vi "HEWH Trigger Below Setpoint.vi"(5 "Station D":T1={"Sequence #"=0.0, "Cycles"=0, "Mode Setting"="", "Flow Rate (GPM)"=0.0, "Temperature (F)"=0.0, "Reset Timer"=FALSE, "Use Temp Decline Method"=FALSE, "Terminate Condition"=enum."C1-Terminate Draw @ Gallon Mark", "Condition Value #1"=0.0, "UE"=FALSE, "LE"=FALSE, "Comp"=FALSE, "Fan"=FALSE, "Test End Time (Sec)"=0.0, "Purge Until Cutout"=FALSE, "Start Conditions"=enum."Heat Source Cutout", "Condition Value #2"=0.0, "Remove Power"=FALSE, "Time"=0.0, "Check Special Cond."=enum."SC2-Check Heat Source (On-C2/Off-C1)", "Condition#"=enum."C1", "Draw Flags"=enum."N/A", "Data Processing Delay (FHD 15sec, UEF 5 Sec)"=0.0, "Test Complete"=FALSE} {"Time" format="%<%H:%M:%S>t"}, 7 "Full Cutout":bool, 8 "Error In":errorcluster, 9 "Array Index":i32, 10 "TC Tree Array":dbl[](array[numeric]), 11 "StationA Setpoint":i32=140 caption="Unit Setpoint") -> (0 "Error Out":errorcluster, 3 "Trigger Draw":bool)   [LabVIEW 2016]
uses:
  Type Definitions/PRAT Test.ctl
  Utility/Save File/File Setup (Public)/Type Definition/Save File HEWH Heating Control Mode.ctl
  Draw Water Specific/Type Definitions/Terminate Draw Conditions.ctl
  Type Definitions/HEWH Start Conditions.ctl
  Draw Water Specific/Type Definitions/Check Special Condtions.ctl
  Draw Water Specific/Type Definitions/HEWH Special Condition Check.ctl
  Type Definitions/HEWH Draw Flag ENUM.ctl
  Utility/Custom Pallet Controls/Custom Pallet String.ctl
  Utility/Type Definitions/UTILITY Notifier.ctl
  Utility/Save File/File Setup.lvlib
panel:
  out "Selected TC Temp (°F)":dbl
  out "Draw Until Temp (°F)":dbl
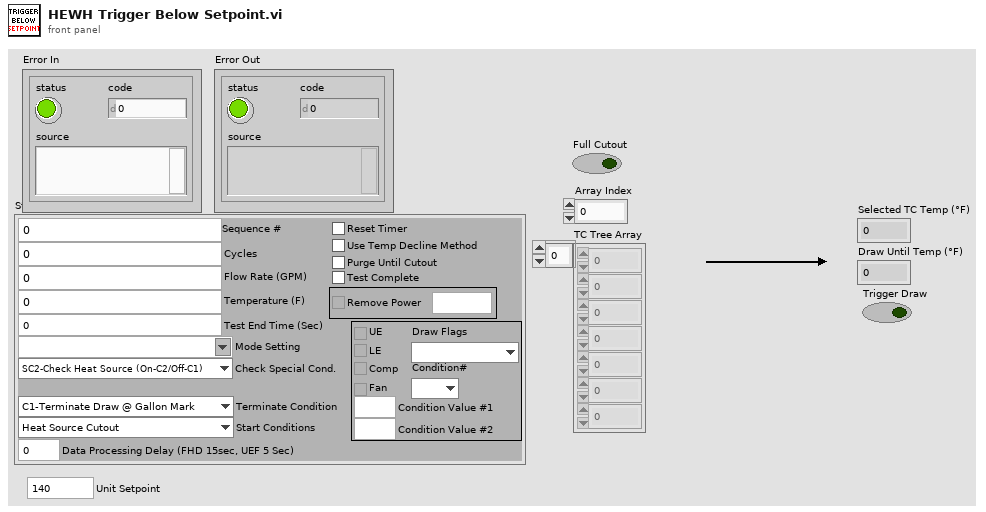
[diagram p1: front panel]
types:
  T1 = typedef "PRAT Test.ctl" = cluster{"Sequence #":dbl, "Cycles":i32, "Mode Setting":T2, "Flow Rate (GPM)":dbl, "Temperature (F)":dbl, "Reset Timer":bool, "Use Temp Decline Method":bool, "Terminate Condition":T3, "Condition Value #1":dbl, "UE":bool, "LE":bool, "Comp":bool, "Fan":bool, "Test End Time (Sec)":dbl, "Purge Until Cutout":bool, "Start Conditions":T4, "Condition Value #2":dbl, "Remove Power":bool, "Time":dbl, "Check Special Cond.":T5, "Condition#":T6, "Draw Flags":T7, "Data Processing Delay (FHD 15sec, UEF 5 Sec)":dbl, "Test Complete":bool}
  T2 = typedef "File Setup.lvlib/Save File HEWH Heating Control Mode.ctl" = string
  T3 = typedef "Terminate Draw Conditions.ctl" = enum16{"C1-Terminate Draw @ Gallon Mark", "C2-Special Last Draw (HU Test)", "C3-RTD Out <=", "C4-Mean Tank Temp <=", "C5-Decrease RTD Out (Deg F)", "C6-Time (Seconds)", "C7-Until Any Heat Source", "C8-Specific Heat Source", "C9-Do Nothing"}
  T4 = typedef "HEWH Start Conditions.ctl" = enum16{"Heat Source Cutout", "At Time (Seconds)", "Every X (Seconds)", "T2 >= X° Below Setpoint", "Seconds From Complete", "Wait for LE & Comp Cutout", "Wait for Comp Cutout", "Wait for LE Cutout", "Wait for UE Cutout"}
  T5 = typedef "Check Special Condtions.ctl" = enum16{"SC1-Do Nothing", "SC2-Check Heat Source (On-C2/Off-C1)", "SC3-Check Skip Condition", "SC4-Check Heat Source ON/Fail"}
  T6 = typedef "HEWH Special Condition Check.ctl" = enum16{"N/A", "C1", "C2", "Reset/Fail", "Skip Draw Sequence"}
  T7 = typedef "HEWH Draw Flag ENUM.ctl" = enum16{"N/A", "None(0)", "Sml(1)", "Med(2)", "SmlMed(3)", "Lrg(4)", "SmlLrg(5)", "MedLrg(6)", "SmlMedLrg(7)"}
  T8 = typedef "Custom Pallet String.ctl" = string
  T9 = typedef "UTILITY Notifier.ctl" = enum16{"Set", "Read", "Release Ref"}
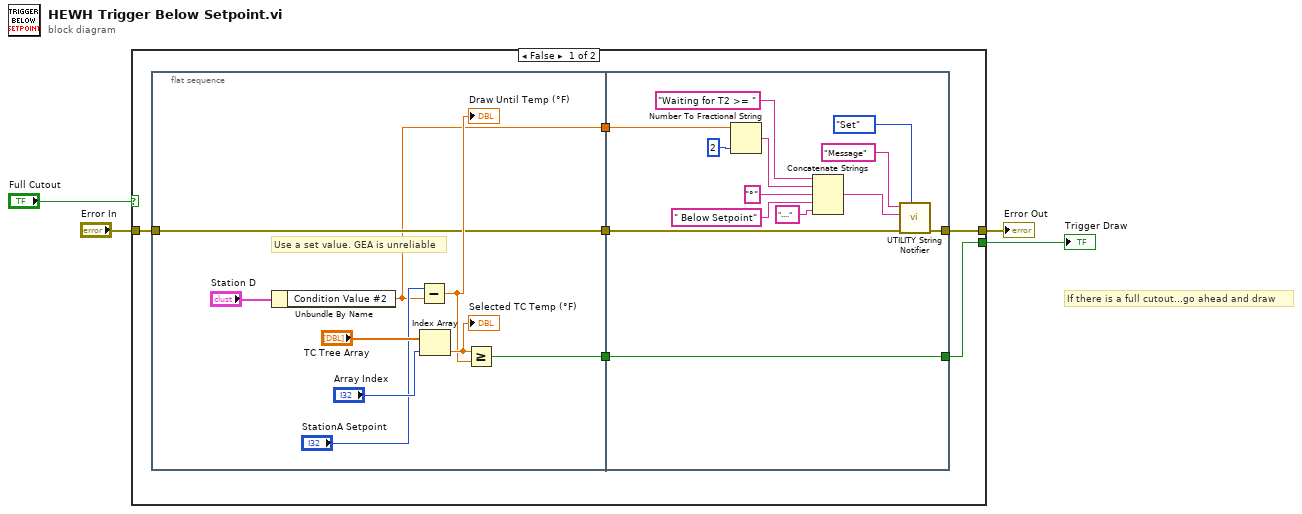
[diagram p0: block diagram]
diagram:
  # "If there is a full cutout...go ahead and draw"
  n1 = case shown="False" "Full Cutout" {
    selector: "Full Cutout" -> [_ w34]
    tunnel: [w10 w34] -> w4
    tunnel: "Error In" -> [w8 w33]
    tunnel: [w6 w33] -> w1
    frame False {
      n2 = flat-sequence {
        tunnel: [w16] -> w9
        tunnel: w8 -> [w12]
        tunnel: [w12] -> w7
        tunnel: [w11] -> w5
        tunnel: [w32] -> w10
        tunnel: w9 -> [w32]
        tunnel: w7 -> [w29]
        tunnel: [w28] -> w6
        tunnel: w5 -> [w26]
        frame #0 {
          # "Use a set value. GEA is unreliable"
          n3 = Unbundle By Name("Station D") -> ("Condition Value #2"=w11:dbl)
          n4 = Subtract(x="StationA Setpoint", y=w11) -> (x-y=w17:dbl)
          "Draw Until Temp (°F)" <- w17
          n5 = Index Array(array="TC Tree Array", index="Array Index") -> (element=w19:dbl)
          "Selected TC Temp (°F)" <- w19
          n6 = Greater Or Equal?(x=w19, y=w17) -> (x >= y?=w16:bool)
        }
        frame #1 {
          n7 = Number To Fractional String(number=w26, precision (6)=i16 2) -> (F-format string=w24:string)  [unwired: 2 in]
          n8 = Concatenate Strings(T8 "Waiting for T2 >= " ("Message"), w24, "°" ("string"), " Below Setpoint" ("string"), T8 "...." ("Message")) -> (w20:string)
          n9 = call "UTILITY String Notifier.vi"("Status"=UTILITY_Notifier."Set", "error in (no error)"=w29, "Set Status"=w20, "name (unnamed)"="Message") -> ("error out"=w28:errorcluster)  [unwired: 6 in, 1 out]
        }
      }
    }
    frame True {
    }
  }
  "Error Out" <- w1
  "Trigger Draw" <- w4
